vi "SenalAudio_a_FrecuenciasDTMF.vi"(3 "time signal in":waveform(dbl)) -> (0 "Min_Frecuencia":dbl, 1 "Max_Frecuencia":dbl)   [LabVIEW 2018]
uses:
  <vilib>/measure/NI_MAPro.lvlib
  <vilib>/measure/matone.llb/Extract Multiple Tone Information 1 Chan.vi
panel:
  in  "Limites_Frecuencias_DTMF_Bajas":T1(array[cluster])=[{"Frecuencia_DTMF"=697.0, "Limite_Inicial"=695.0, "Limite_Final"=699.0}, {"Frecuencia_DTMF"=770.0, "Limite_Inicial"=768.0, "Limite_Final"=772.0}, {"Frecuencia_DTMF"=852.0, "Limite_Inicial"=850.0, "Limite_Final"=854.0}, {"Frecuencia_DTMF"=941.0, "Limite_Inicial"=939.0, "Limite_Final"=943.0}]
  in  "Limites_Frecuencias_DTMF_Altas":T1(array[cluster])=[{"Frecuencia_DTMF"=1209.0, "Limite_Inicial"=1207.0, "Limite_Final"=1211.0}, {"Frecuencia_DTMF"=1336.0, "Limite_Inicial"=1334.0, "Limite_Final"=1338.0}, {"Frecuencia_DTMF"=1477.0, "Limite_Inicial"=1475.0, "Limite_Final"=1479.0}, {"Frecuencia_DTMF"=1633.0, "Limite_Inicial"=1631.0, "Limite_Final"=1635.0}]
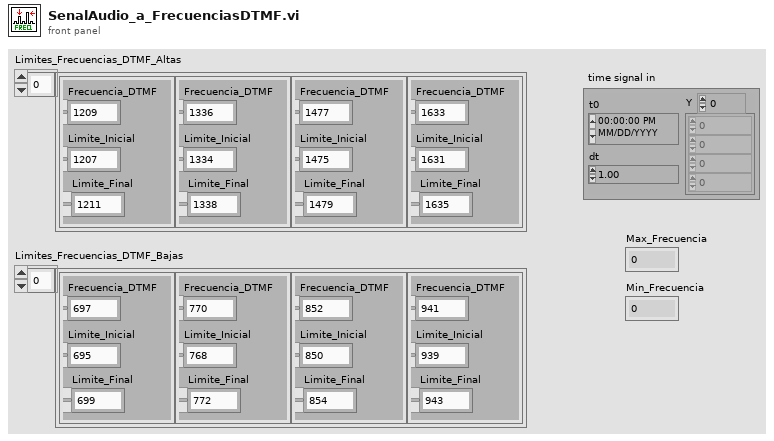
[diagram p1: front panel]
types:
  T1 = cluster{"Frecuencia_DTMF":dbl, "Limite_Inicial":dbl, "Limite_Final":dbl}[]
  T2 = cluster{"detected frequency":dbl, "detected amplitude":dbl, "detected phase (deg)":dbl}[]
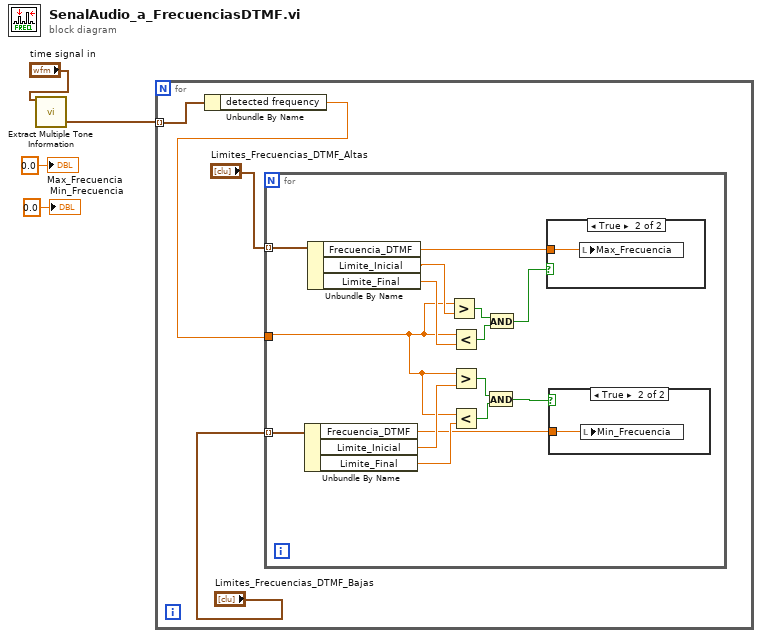
[diagram p0: block diagram]
diagram:
  n1 = call-poly <vilib>:"Extract Multiple Tone Information.vi"("time signal in"="time signal in") -> ("multiple tone information"=w1:T2)  [unwired: 12 in, 2 out]
  n2 = for {
    tunnel: w1 -> [w6] mode=indexing
    n3 = Unbundle By Name(w6) -> ("detected frequency"=w5:dbl)
    n4 = for {
      tunnel: "Limites_Frecuencias_DTMF_Bajas" -> [w22] mode=indexing
      tunnel: "Limites_Frecuencias_DTMF_Altas" -> [w23] mode=indexing
      tunnel: w5 -> [w18]
      n5 = Unbundle By Name(w22) -> ("Frecuencia_DTMF"=w9:dbl, "Limite_Inicial"=w19:dbl, "Limite_Final"=w17:dbl)
      n6 = Unbundle By Name(w23) -> ("Frecuencia_DTMF"=w13:dbl, "Limite_Inicial"=w21:dbl, "Limite_Final"=w20:dbl)
      n7 = Greater?(x=w18, y=w21) -> (0:w16:bool)
      n8 = Less?(x=w18, y=w20) -> (x < y?=w15:bool)
      n9 = Greater?(x=w18, y=w19) -> (0:w12:bool)
      n10 = Less?(x=w18, y=w17) -> (x < y?=w11:bool)
      n11 = And(x=w12, y=w11) -> (x .and. y?=w10:bool)
      n12 = And(x=w16, y=w15) -> (x .and. y?=w14:bool)
      n13 = case shown="True" w14 {
        tunnel: w13 -> [_ w25]
        frame False {
        }
        frame True {
          n14 = local write "Max_Frecuencia"(w25) -> ()
        }
      }
      n15 = case shown="True" w10 {
        tunnel: w9 -> [_ w24]
        frame False {
        }
        frame True {
          n16 = local write "Min_Frecuencia"(w24) -> ()
        }
      }
    }
  }
  "Max_Frecuencia" <- 0.0 ("Max_Frecuencia")
  "Min_Frecuencia" <- 0.0 ("Min_Frecuencia")
